vi "ShutDownTimingDIO_ScannerStage.vi"(0 "task out 7":refnum<k21>, 1 "error IO":errorcluster, 2 "task out 2":refnum<k21>, 3 "task out 3":refnum<k21>, 5 "task out 5":refnum<k21>, 8 "task out 9":refnum<k21>, 9 "task out":refnum<k21>, 11 "task out 10":refnum<k21>, 17 "task out 6":refnum<k21>, 19 "task out 4":refnum<k21>) -> (15 "error out":errorcluster)   [LabVIEW 2011]
uses:
  <vilib>/Utility/error.llb/DialogType.ctl
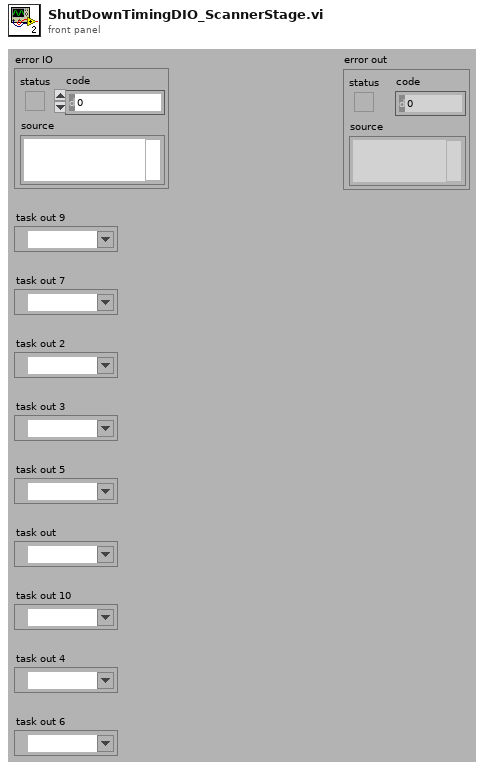
[diagram p1: front panel]
types:
  T1 = typedef "DialogType.ctl" = u16
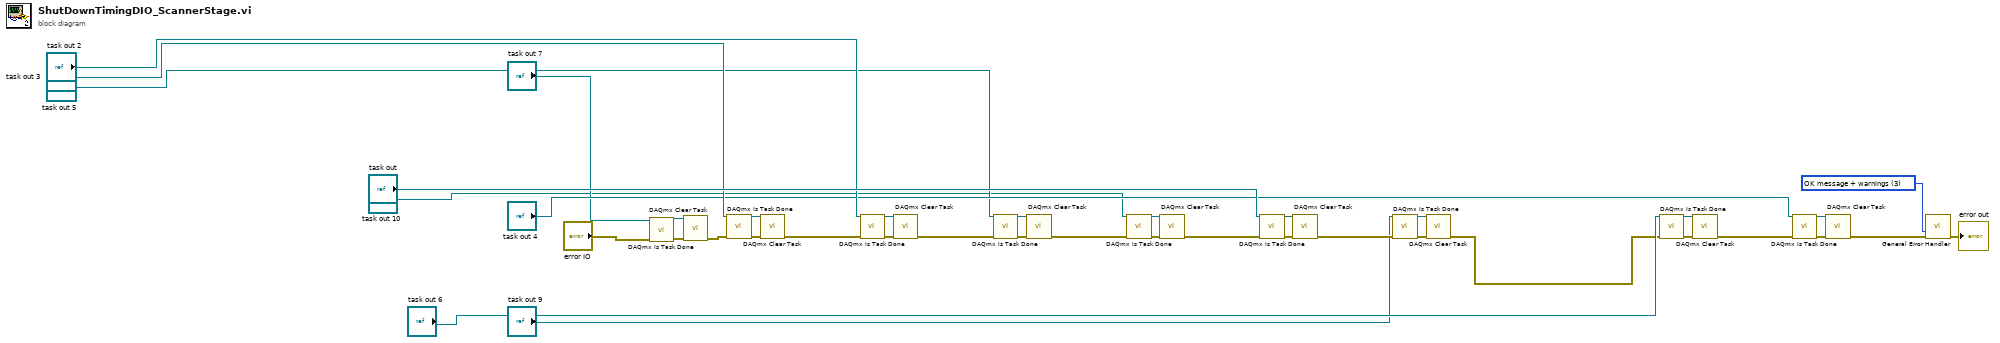
[diagram p0: block diagram]
diagram:
  w3 = T1 3 items=["no dialog", "OK message", "continue or stop message", "OK message + warnings", "continue/stop + warnings"] ("type of dialog (OK msg:1)")
  n1 = call <vilib>:"DAQmx Is Task Done.vi"("task/channels in"="task out 7", "error in"="error IO") -> ("task out"=w2:refnum<k21>, "error out"=w4:errorcluster)  [unwired: 11 in, 1 out]
  n2 = call <vilib>:"DAQmx Clear Task.vi"("task in"=w2, "error in"=w4) -> ("error out"=w25:errorcluster)  [unwired: 13 in]
  n3 = call <vilib>:"DAQmx Is Task Done.vi"("task/channels in"="task out 3", "error in"=w25) -> ("task out"=w23:refnum<k21>, "error out"=w21:errorcluster)  [unwired: 11 in, 1 out]
  n4 = call <vilib>:"DAQmx Clear Task.vi"("task in"=w23, "error in"=w21) -> ("error out"=w24:errorcluster)  [unwired: 13 in]
  n5 = call <vilib>:"DAQmx Is Task Done.vi"("task/channels in"="task out 2", "error in"=w24) -> ("task out"=w29:refnum<k21>, "error out"=w22:errorcluster)  [unwired: 11 in, 1 out]
  n6 = call <vilib>:"DAQmx Clear Task.vi"("task in"=w29, "error in"=w22) -> ("error out"=w26:errorcluster)  [unwired: 13 in]
  n7 = call <vilib>:"DAQmx Is Task Done.vi"("task/channels in"="task out 5", "error in"=w26) -> ("task out"=w18:refnum<k21>, "error out"=w17:errorcluster)  [unwired: 11 in, 1 out]
  n8 = call <vilib>:"DAQmx Clear Task.vi"("task in"=w18, "error in"=w17) -> ("error out"=w37:errorcluster)  [unwired: 13 in]
  n9 = call <vilib>:"DAQmx Is Task Done.vi"("task/channels in"="task out 10", "error in"=w37) -> ("task out"=w6:refnum<k21>, "error out"=w7:errorcluster)  [unwired: 11 in, 1 out]
  n10 = call <vilib>:"DAQmx Clear Task.vi"("task in"=w6, "error in"=w7) -> ("error out"=w31:errorcluster)  [unwired: 13 in]
  n11 = call <vilib>:"DAQmx Is Task Done.vi"("task/channels in"="task out", "error in"=w31) -> ("task out"=w33:refnum<k21>, "error out"=w30:errorcluster)  [unwired: 11 in, 1 out]
  n12 = call <vilib>:"DAQmx Clear Task.vi"("task in"=w33, "error in"=w30) -> ("error out"=w32:errorcluster)  [unwired: 13 in]
  n13 = call <vilib>:"DAQmx Is Task Done.vi"("task/channels in"="task out 9", "error in"=w32) -> ("task out"=w8:refnum<k21>, "error out"=w5:errorcluster)  [unwired: 11 in, 1 out]
  n14 = call <vilib>:"DAQmx Clear Task.vi"("task in"=w8, "error in"=w5) -> ("error out"=w1:errorcluster)  [unwired: 13 in]
  n15 = call <vilib>:"DAQmx Is Task Done.vi"("task/channels in"="task out 6", "error in"=w1) -> ("task out"=w14:refnum<k21>, "error out"=w12:errorcluster)  [unwired: 11 in, 1 out]
  n16 = call <vilib>:"DAQmx Clear Task.vi"("task in"=w14, "error in"=w12) -> ("error out"=w35:errorcluster)  [unwired: 13 in]
  n17 = call <vilib>:"DAQmx Is Task Done.vi"("task/channels in"="task out 4", "error in"=w35) -> ("task out"=w16:refnum<k21>, "error out"=w15:errorcluster)  [unwired: 11 in, 1 out]
  n18 = call <vilib>:"DAQmx Clear Task.vi"("task in"=w16, "error in"=w15) -> ("error out"=w39:errorcluster)  [unwired: 13 in]
  n19 = call <vilib>:"General Error Handler.vi"("type of dialog (OK msg:1)"=w3, "error in (no error)"=w39) -> ("error out"=→"error out":errorcluster)  [unwired: 9 in, 4 out]
